vi "TDM_Abhishek_Barla.vi"() -> ()   [LabVIEW 2015]
uses:
  <vilib>/Waveform/DWDTOps.llb/DWDT Analog to Digital.vi
  <vilib>/Waveform/DWDTOps.llb/DWDT Digital to Binary U32.vi
  <vilib>/Waveform/DWDTOps.llb/DWDT Binary U32 to Digital.vi
  <vilib>/Waveform/DWDTOps.llb/DWDT Digital to Analog.vi
  <vilib>/sound2/lvsound2.llb/Sound Output Set Volume (Single).vi
panel:
  in  "Set Output Sound Volume":dbl(slide) scale=0.0..10.0
  in  "Waveform 7 or Waveform 8":enum16{"Waveform 7", "Waveform 8"}(ring) caption="Which Audio file would you want to play?"
  out "Waveform Graph 8":waveform(dbl)(graph)
  out "Waveform Graph 7":waveform(dbl)(graph)
  out "Waveform Graph 6":waveform(dbl)(graph)
  out "Waveform Graph 5":waveform(dbl)(graph)
  out "Waveform Graph 4":waveform(dbl)(graph)
  out "Digital Signal for Second File":digitalwaveform(graph)
  out "Digital Signal for First File":digitalwaveform(graph)
  in  "?":path
  in  "?":path
  out "File Data 2":waveform(dbl)[](graph)
  in  "Number of Samples 2":i32=-1
  out "File Data":waveform(dbl)[](graph)
  in  "Number of Samples":i32=-1
  out "Waveform Graph 3":dynamicdata(graph)
  in  "Type of Waveform 3":T1(ring)
  out "Waveform Graph 2":dynamicdata(graph)
  in  "Type of Waveform 2":T1(ring)
  out "Waveform Graph 1":dynamicdata(graph)
  in  "Type of Waveform Type of Waveform1":T1(ring) caption="Type of Waveform 1"
  # "Virtual Instrumentation Lab - Midterm Project - Fall 2015 - Ali_Aldhaheri"
  # "Please Select the First .wav File"
  # "Please Select the Second .wav File"
  # "Analog \n Signal"
  # "Analog Signal"
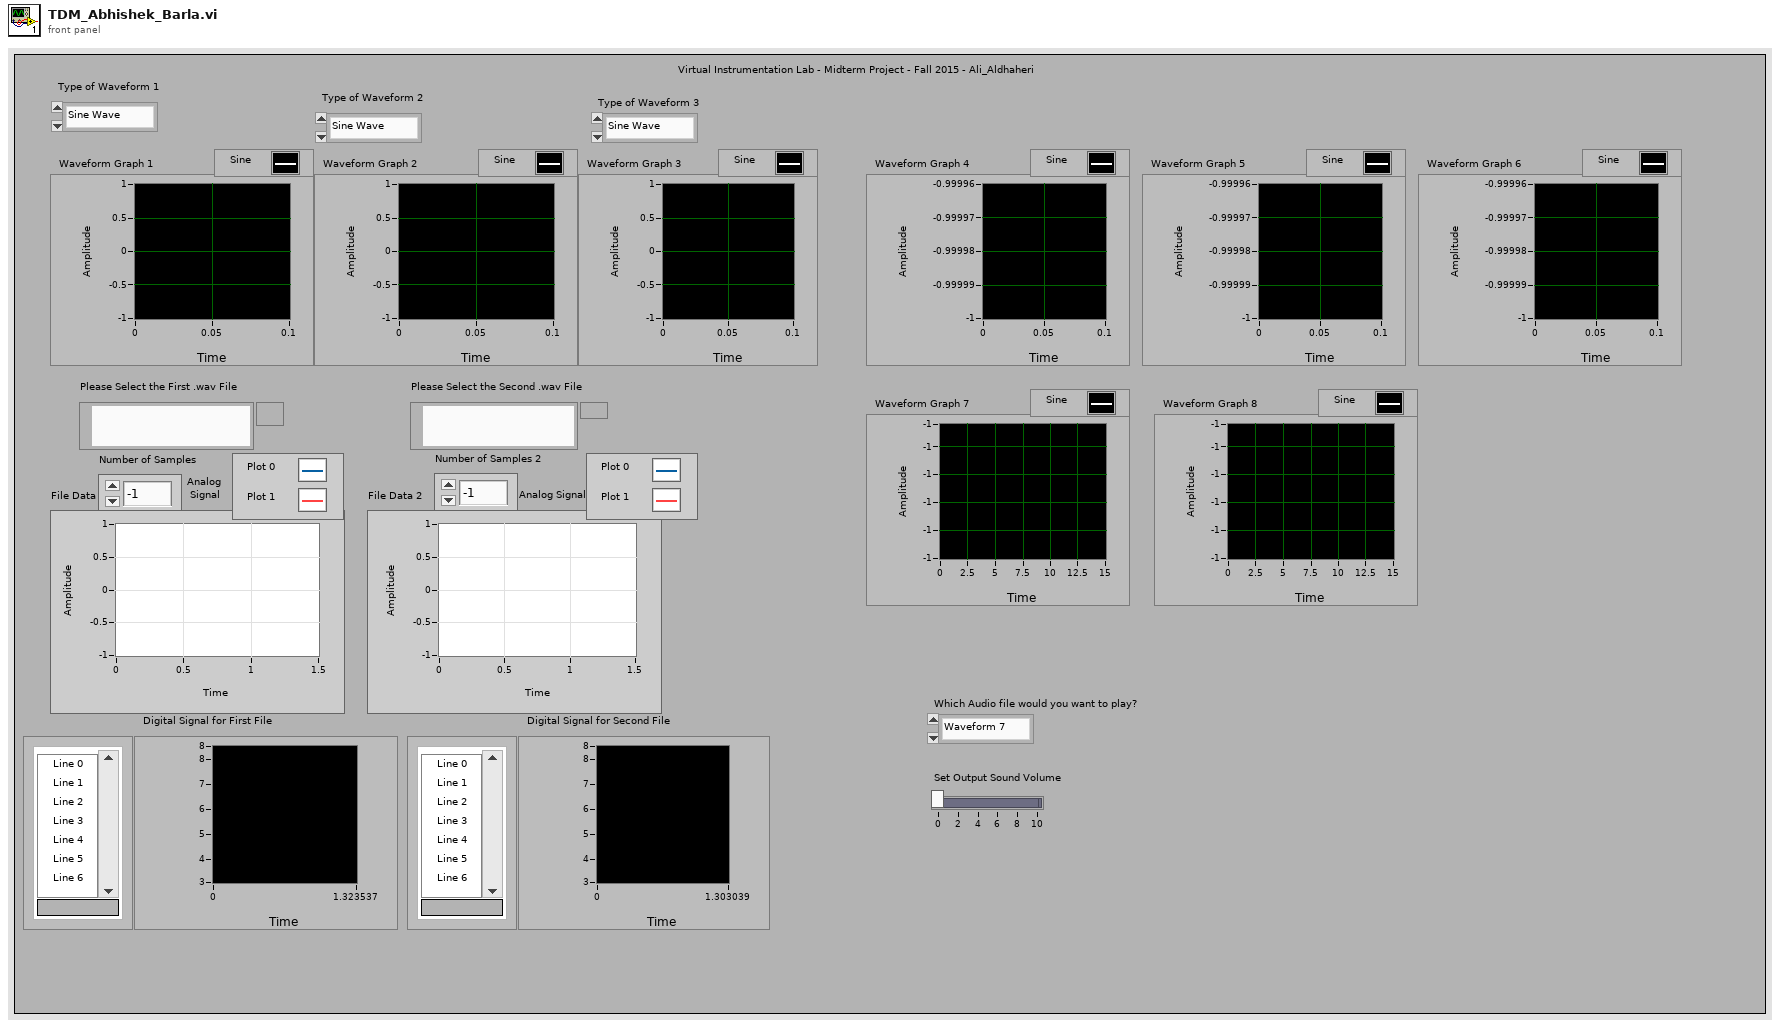
[diagram p1: front panel]
types:
  T1 = enum16{"Sine Wave", "Square Wave", "Saw Tooth Wave", "Triangular Wave", "DC Wave"}
  T2 = typedef "Sound Output Task ID.ctl" = u32
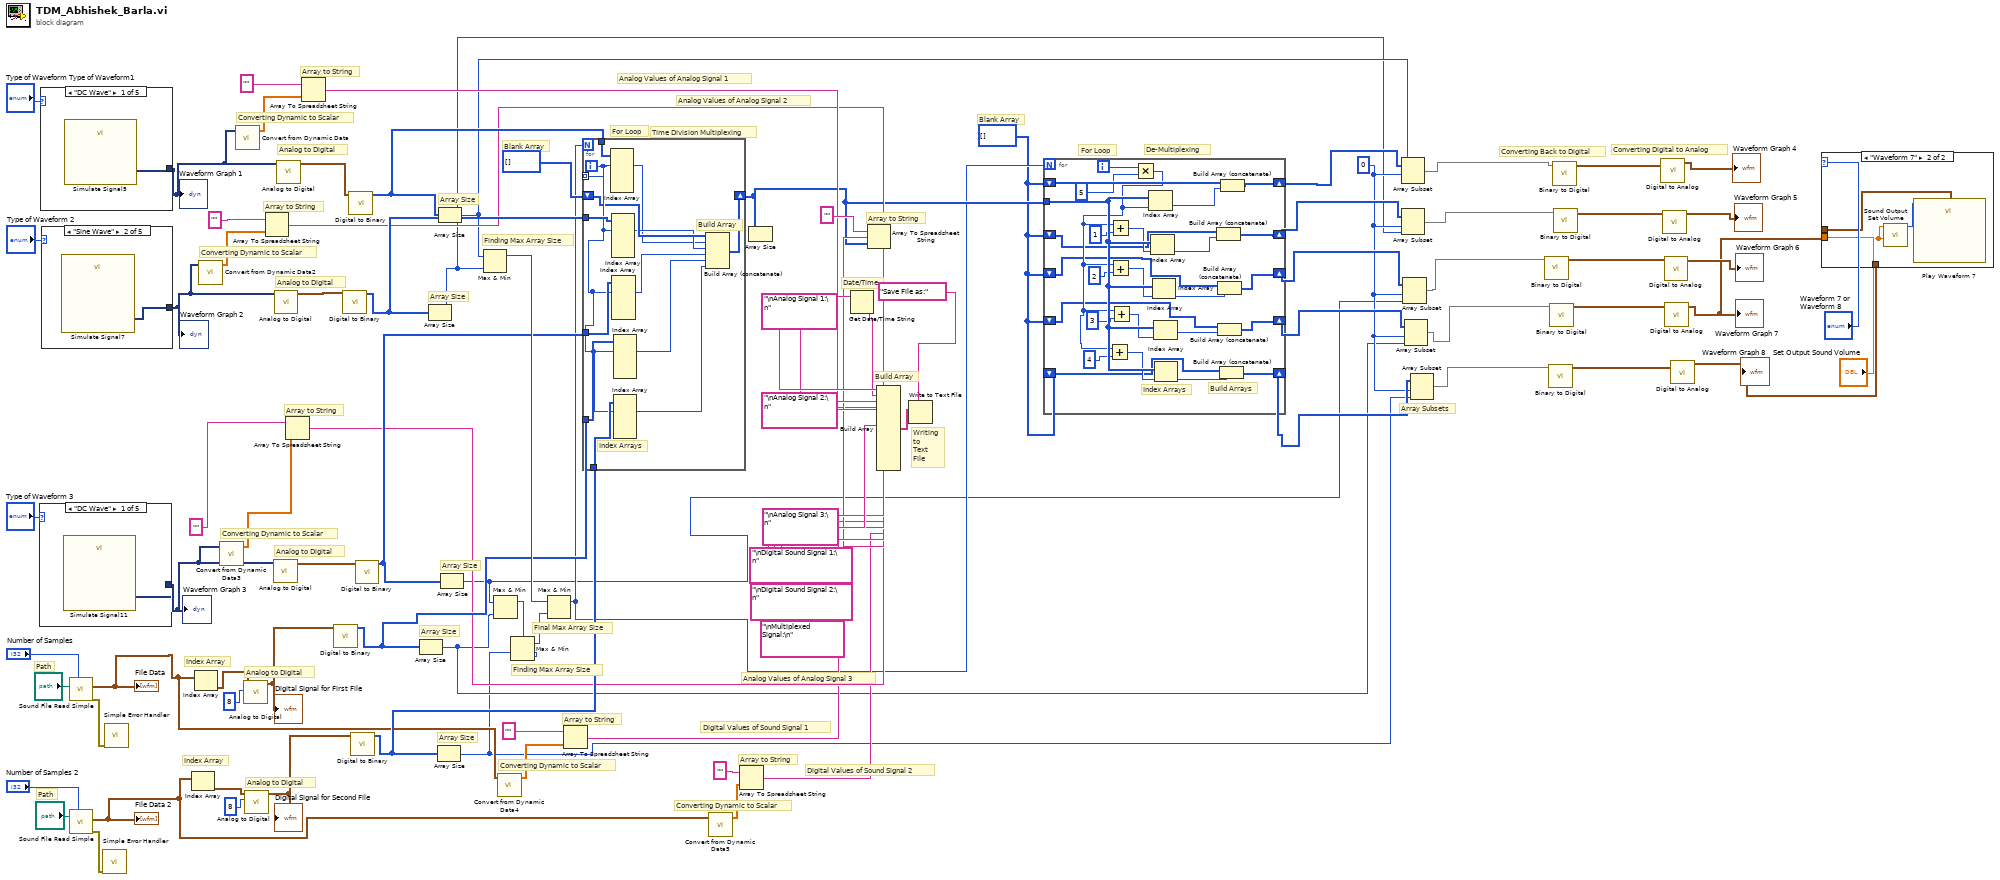
[diagram p0: block diagram]
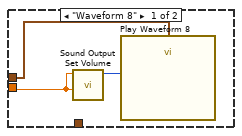
[diagram p2: hidden frame]
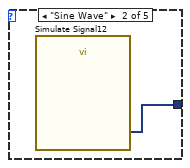
[diagram p3: hidden frame]
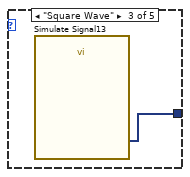
[diagram p4: hidden frame]
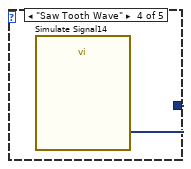
[diagram p5: hidden frame]
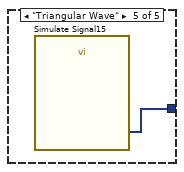
[diagram p6: hidden frame]
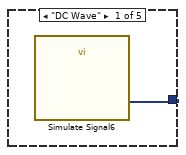
[diagram p7: hidden frame]
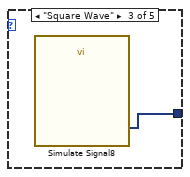
[diagram p8: hidden frame]
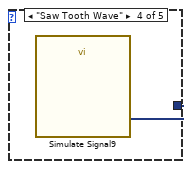
[diagram p9: hidden frame]
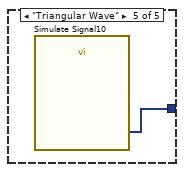
[diagram p10: hidden frame]
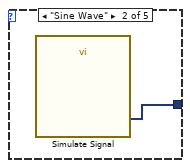
[diagram p11: hidden frame]
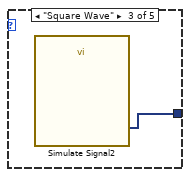
[diagram p12: hidden frame]
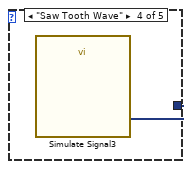
[diagram p13: hidden frame]
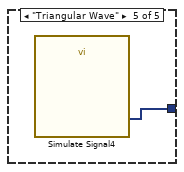
[diagram p14: hidden frame]
diagram:
  w23 = 0
  w29 = i32[] []
  # "Converting Digital to Analog"
  # "Converting Back to Digital"
  # "Array Subsets"
  # "Blank Array"
  # "Digital Values of Sound Signal 2"
  # "Digital Values of Sound Signal 1"
  # "Converting Dynamic to Scalar"
  # "Array to String"
  # "Converting Dynamic to Scalar"
  # "Array to String"
  # "Analog Values of Analog Signal 3"
  # "Converting Dynamic to Scalar"
  # "Array to String"
  # "Analog Values of Analog Signal 2"
  # "Analog Values of Analog Signal 1"
  # "Converting Dynamic to Scalar"
  # "Array to String"
  # "Converting Dynamic to Scalar"
  # "Array to String"
  # "Build Array"
  # "Array to String"
  # "Date/Time"
  # "Writing\nto \nText \nFile"
  # "De-Multiplexing"
  # "For Loop"
  # "Blank Array"
  # "Final Max Array Size"
  # "Finding Max Array Size"
  # "Finding Max Array Size"
  # "Array Size"
  # "Array Size"
  # "Array Size"
  # "Array Size"
  # "Array Size"
  # "For Loop"
  # "Analog to Digital"
  # "Analog to Digital"
  # "Analog to Digital"
  # "Time Division Multiplexing"
  # "Index Array"
  # "Index Array"
  # "Path"
  # "Path"
  # "Analog to Digital"
  # "Analog to Digital"
  n1 = case shown="\"DC Wave\"" "Type of Waveform 3" {
    tunnel: [w91 w92 w93 w94 w95] -> w41
    frame "DC Wave" {
      n2 = call "Simulate Signal11"() -> ("DC"=w91:dynamicdata)  [unwired: 14 in, 1 out]
    }
    frame "Sine Wave" {
      n3 = call "Simulate Signal12"() -> ("Sine"=w92:dynamicdata)  [unwired: 14 in, 1 out]
    }
    frame "Square Wave" {
      n4 = call "Simulate Signal13"() -> ("Square"=w93:dynamicdata)  [unwired: 14 in, 1 out]
    }
    frame "Saw Tooth Wave" {
      n5 = call "Simulate Signal14"() -> ("Sawtooth"=w94:dynamicdata)  [unwired: 14 in, 1 out]
    }
    frame "Triangular Wave" {
      n6 = call "Simulate Signal15"() -> ("Triangle"=w95:dynamicdata)  [unwired: 14 in, 1 out]
    }
  }
  "Waveform Graph 3" <- w41
  n7 = case shown="\"DC Wave\"" "Type of Waveform Type of Waveform1" {
    tunnel: [w96 w97 w98 w99 w100] -> w50
    frame "DC Wave" {
      n8 = call "Simulate Signal5"() -> ("DC"=w96:dynamicdata)  [unwired: 14 in, 1 out]
    }
    frame "Sine Wave" {
      n9 = call "Simulate Signal"() -> ("Sine"=w97:dynamicdata)  [unwired: 14 in, 1 out]
    }
    frame "Square Wave" {
      n10 = call "Simulate Signal2"() -> ("Square"=w98:dynamicdata)  [unwired: 14 in, 1 out]
    }
    frame "Saw Tooth Wave" {
      n11 = call "Simulate Signal3"() -> ("Sawtooth"=w99:dynamicdata)  [unwired: 14 in, 1 out]
    }
    frame "Triangular Wave" {
      n12 = call "Simulate Signal4"() -> ("Triangle"=w100:dynamicdata)  [unwired: 14 in, 1 out]
    }
  }
  "Waveform Graph 1" <- w50
  n13 = case shown="\"Sine Wave\"" "Type of Waveform 2" {
    tunnel: [w101 w102 w103 w104 w105] -> w45
    frame "DC Wave" {
      n14 = call "Simulate Signal6"() -> ("DC"=w101:dynamicdata)  [unwired: 14 in, 1 out]
    }
    frame "Sine Wave" {
      n15 = call "Simulate Signal7"() -> ("Sine"=w102:dynamicdata)  [unwired: 14 in, 1 out]
    }
    frame "Square Wave" {
      n16 = call "Simulate Signal8"() -> ("Square"=w103:dynamicdata)  [unwired: 14 in, 1 out]
    }
    frame "Saw Tooth Wave" {
      n17 = call "Simulate Signal9"() -> ("Sawtooth"=w104:dynamicdata)  [unwired: 14 in, 1 out]
    }
    frame "Triangular Wave" {
      n18 = call "Simulate Signal10"() -> ("Triangle"=w105:dynamicdata)  [unwired: 14 in, 1 out]
    }
  }
  "Waveform Graph 2" <- w45
  n19 = call <vilib>:"Sound File Read Simple.vi"("number of samples/ch (-1: all)"="Number of Samples", "path"="?") -> ("error out"=w86:errorcluster, "data"=w35:waveform(dbl)[])  [unwired: 6 in, 2 out]
  "File Data" <- w35
  n20 = call <vilib>:"Sound File Read Simple.vi"("number of samples/ch (-1: all)"="Number of Samples 2", "path"="?") -> ("error out"=w84:errorcluster, "data"=w32:waveform(dbl)[])  [unwired: 6 in, 2 out]
  "File Data 2" <- w32
  n21 = call <vilib>:"Simple Error Handler.vi"("error in (no error)"=w84) -> ()  [unwired: 4 in, 5 out]
  n22 = call <vilib>:"Simple Error Handler.vi"("error in (no error)"=w86) -> ()  [unwired: 4 in, 5 out]
  n23 = Index Array(array=w32) -> (element=w80:waveform(dbl))  [unwired: 1 in]
  n24 = Index Array(array=w35) -> (element=w81:waveform(dbl))  [unwired: 1 in]
  n25 = call "Convert from Dynamic Data2"("Dynamic Data Type"=w45) -> ("Array"=w47:dbl[])  [unwired: 3 in]
  n26 = call "Convert from Dynamic Data3"("Dynamic Data Type"=w41) -> ("Array"=w42:dbl[])  [unwired: 3 in]
  n27 = call "Convert from Dynamic Data"("Dynamic Data Type"=w50) -> ("Array"=w49:dbl[])  [unwired: 3 in]
  n28 = call-poly <vilib>:"Analog to Digital.vi"("resolution (16 bit)"=8, "analog waveform"=w81) -> ("digital waveform"=w74:digitalwaveform)  [unwired: 6 in, 3 out]
  "Digital Signal for First File" <- w74
  n29 = call-poly <vilib>:"Analog to Digital.vi"("resolution (16 bit)"=8, "analog waveform"=w80) -> ("digital waveform"=w75:digitalwaveform)  [unwired: 6 in, 3 out]
  "Digital Signal for Second File" <- w75
  n30 = Array To Spreadsheet String(array=w47, 3:"") -> (spreadsheet string=w44:string)  [unwired: 1 in]
  n31 = call-poly <vilib>:"Analog to Digital.vi"("analog waveform"=w41) -> ("digital waveform"=w73:digitalwaveform)  [unwired: 7 in, 3 out]
  n32 = call-poly <vilib>:"Analog to Digital.vi"("analog waveform"=w45) -> ("digital waveform"=w76:digitalwaveform)  [unwired: 7 in, 3 out]
  n33 = call-poly <vilib>:"Analog to Digital.vi"("analog waveform"=w50) -> ("digital waveform"=w77:digitalwaveform)  [unwired: 7 in, 3 out]
  n34 = Array To Spreadsheet String(array=w42, 3:"") -> (spreadsheet string=w40:string)  [unwired: 1 in]
  n35 = Array To Spreadsheet String(array=w49, 3:"") -> (spreadsheet string=w48:string)  [unwired: 1 in]
  n36 = call-poly <vilib>:"Digital to Binary.vi"("digital waveform"=w74) -> ("binary array"=w64:u32[])  [unwired: 9 in, 1 out]
  n37 = call-poly <vilib>:"Digital to Binary.vi"("digital waveform"=w76) -> ("binary array"=w67:u32[])  [unwired: 9 in, 1 out]
  n38 = call-poly <vilib>:"Digital to Binary.vi"("digital waveform"=w77) -> ("binary array"=w68:u32[])  [unwired: 9 in, 1 out]
  n39 = call-poly <vilib>:"Digital to Binary.vi"("digital waveform"=w75) -> ("binary array"=w65:u32[])  [unwired: 9 in, 1 out]
  n40 = call-poly <vilib>:"Digital to Binary.vi"("digital waveform"=w73) -> ("binary array"=w66:u32[])  [unwired: 9 in, 1 out]
  n41 = Array Size(array=w64) -> (size(s)=w19:i32)
  n42 = Array Size(array=w67) -> (size(s)=w21:i32)
  n43 = Array Size(array=w65) -> (size(s)=w18:i32)
  n44 = Array Size(array=w68) -> (size(s)=w22:i32)
  n45 = Array Size(array=w66) -> (size(s)=w20:i32)
  n46 = Max & Min(x=w22, y=w21) -> (max(x,y)=w70:i32)  [unwired: 1 out]
  n47 = Max & Min(x=w20, y=w19) -> (max(x,y)=w72:i32)  [unwired: 1 out]
  n48 = call "Convert from Dynamic Data4"("Dynamic Data Type"=w35) -> ("Array"=w38:dbl[])  [unwired: 3 in]
  n49 = Max & Min(x=w72, y=w18) -> (max(x,y)=w71:i32)  [unwired: 1 out]
  n50 = Max & Min(x=w70, y=w71) -> (max(x,y)=w30:i32)  [unwired: 1 out]
  n51 = Array To Spreadsheet String(array=w38, 3:"") -> (spreadsheet string=w34:string)  [unwired: 1 in]
  n52 = for {
    N: w30 -> [_]
    tunnel: w68 -> [w118]
    tunnel: w67 -> [w117]
    tunnel: w66 -> [w116]
    tunnel: w64 -> [w115]
    tunnel: w65 -> [w114]
    shift-right: [w112] -> w31
    shift-left: i32[] [] -> [w111]
    tunnel: [w113] -> _ mode=indexing
    i -> [w113]
    # "Build Array"
    # "Index Arrays"
    n53 = Index Array(array=w118, index #1=w113) -> (element #1=w106:u32)  [unwired: 4 in, 4 out]
    n54 = Index Array(array=w117, index #1=w113) -> (element #1=w107:u32)  [unwired: 4 in, 4 out]
    n55 = Index Array(array=w116, index #1=w113) -> (element #1=w108:u32)  [unwired: 4 in, 4 out]
    n56 = Index Array(array=w115, index #1=w113) -> (element #1=w109:u32)  [unwired: 4 in, 4 out]
    n57 = Index Array(array=w114, index #1=w113) -> (element #1=w110:u32)  [unwired: 4 in, 4 out]
    n58 = Build Array (concatenate)(w111, w106, w107, w108, w109, w110) -> (w112:u32[])
  }
  n59 = call "Convert from Dynamic Data5"("Dynamic Data Type"=w32) -> ("Array"=w36:dbl[])  [unwired: 3 in]
  n60 = Array To Spreadsheet String(array=w36, 3:"") -> (spreadsheet string=w33:string)  [unwired: 1 in]
  n61 = Array Size(array=w31) -> ()  [unwired: 1 out]
  n62 = Get Date/Time String() -> (date string=w62:string, time string=w61:string)  [unwired: 3 in]
  n63 = Array To Spreadsheet String(array=w31, 3:"") -> (spreadsheet string=w52:string)  [unwired: 1 in]
  n64 = Build Array(w62, w61, "\nAnalog Signal 1:\n", w48, "\nAnalog Signal 2:\n", w44, "\nAnalog Signal 3:\n", w40, "\nDigital Sound Signal 1:\n", w34, "\nDigital Sound Signal 2:\n", w33, "\nMultiplexed Signal:\n", w52) -> (w60:string[])
  n65 = Write to Text File(prompt (Choose or enter file path)="Save File as:", text=w60) -> ()  [unwired: 2 in, 3 out]
  n66 = for {
    N: w30 -> [_]
    tunnel: w31 -> [w144]
    shift-right: [w145] -> w28
    shift-left: w29 -> [w126]
    shift-right: [w138] -> w24
    shift-left: w29 -> [w122]
    shift-right: [w137] -> w27
    shift-left: w29 -> [w121]
    shift-right: [w136] -> w26
    shift-left: w29 -> [w120]
    shift-right: [w135] -> w25
    shift-left: w29 -> [w119]
    i -> [w125]
    # "Build Arrays"
    # "Index Arrays"
    n67 = Multiply(x=w125, y=5) -> (x*y=w124:i32)
    n68 = Add(x=w124, y=4) -> (x+y=w128:i32)
    n69 = Add(x=w124, y=1) -> (x+y=w133:i32)
    n70 = Add(x=w124, y=2) -> (x+y=w131:i32)
    n71 = Add(x=w124, y=3) -> (x+y=w127:i32)
    n72 = Index Array(array=w144, index=w124) -> (element=w143:u32)
    n73 = Index Array(array=w144, index=w133) -> (element=w139:u32)
    n74 = Index Array(array=w144, index=w131) -> (element=w140:u32)
    n75 = Index Array(array=w144, index=w127) -> (element=w141:u32)
    n76 = Index Array(array=w144, index=w128) -> (element=w142:u32)
    n77 = Build Array (concatenate)(w122, w139) -> (w138:u32[])
    n78 = Build Array (concatenate)(w121, w140) -> (w137:u32[])
    n79 = Build Array (concatenate)(w120, w141) -> (w136:u32[])
    n80 = Build Array (concatenate)(w119, w142) -> (w135:u32[])
    n81 = Build Array (concatenate)(w126, w143) -> (w145:u32[])
  }
  n82 = Array Subset(array=w28, index=w23, length=w22) -> (w17:u32[])
  n83 = Array Subset(array=w24, index=w23, length=w21) -> (w13:u32[])
  n84 = Array Subset(array=w27, index=w23, length=w20) -> (w14:u32[])
  n85 = Array Subset(array=w26, index=w23, length=w19) -> (w15:u32[])
  n86 = Array Subset(array=w25, index=w23, length=w18) -> (w16:u32[])
  n87 = call-poly <vilib>:"Binary to Digital.vi"("binary array"=w14) -> ("digital waveform"=w9:digitalwaveform)  [unwired: 9 in, 1 out]
  n88 = call-poly <vilib>:"Binary to Digital.vi"("binary array"=w16) -> ("digital waveform"=w11:digitalwaveform)  [unwired: 9 in, 1 out]
  n89 = call-poly <vilib>:"Binary to Digital.vi"("binary array"=w15) -> ("digital waveform"=w10:digitalwaveform)  [unwired: 9 in, 1 out]
  n90 = call-poly <vilib>:"Binary to Digital.vi"("binary array"=w17) -> ("digital waveform"=w12:digitalwaveform)  [unwired: 9 in, 1 out]
  n91 = call-poly <vilib>:"Binary to Digital.vi"("binary array"=w13) -> ("digital waveform"=w8:digitalwaveform)  [unwired: 9 in, 1 out]
  n92 = call-poly <vilib>:"Digital to Analog.vi"("digital waveform"=w12) -> ("analog waveform"=→"Waveform Graph 4":waveform(dbl))  [unwired: 7 in, 3 out]
  n93 = call-poly <vilib>:"Digital to Analog.vi"("digital waveform"=w8) -> ("analog waveform"=→"Waveform Graph 5":waveform(dbl))  [unwired: 7 in, 3 out]
  n94 = call-poly <vilib>:"Digital to Analog.vi"("digital waveform"=w9) -> ("analog waveform"=→"Waveform Graph 6":waveform(dbl))  [unwired: 7 in, 3 out]
  n95 = call-poly <vilib>:"Digital to Analog.vi"("digital waveform"=w10) -> ("analog waveform"=w4:waveform(dbl))  [unwired: 7 in, 3 out]
  "Waveform Graph 7" <- w4
  n96 = call-poly <vilib>:"Digital to Analog.vi"("digital waveform"=w11) -> ("analog waveform"=w1:waveform(dbl))  [unwired: 7 in, 3 out]
  "Waveform Graph 8" <- w1
  n97 = case shown="\"Waveform 7\"" "Waveform 7 or Waveform 8" {
    tunnel: w4 -> [w148 w151]
    tunnel: w1 -> [_ _]
    tunnel: "Set Output Sound Volume" -> [w146 w149]
    frame "Waveform 8" {
      n98 = call-poly <vilib>:"Sound Output Set Volume.vi"("volume"=w146, "task ID"=w146) -> ("task ID out"=w147:T2)  [unwired: 8 in, 1 out]
      n99 = call "Play Waveform 8"("Device"=w147, "Data"=w148) -> ()  [unwired: 17 in, 1 out]
    }
    frame "Waveform 7" {
      n100 = call-poly <vilib>:"Sound Output Set Volume.vi"("volume"=w149, "task ID"=w149) -> ("task ID out"=w150:T2)  [unwired: 8 in, 1 out]
      n101 = call "Play Waveform 7"("Device"=w150, "Data"=w151) -> ()  [unwired: 17 in, 1 out]
    }
  }
